vi "combinate.vi"(8 "error in (no error)":errorcluster caption="错误输入（无错误）", 11 "HJ212 输入":refnum<class "HJ212.lvclass">) -> (0 "error out":errorcluster caption="错误输出", 3 "HJ212 输出":refnum<class "HJ212.lvclass">)   [LabVIEW 2016, in "中水三立SQL数据传输.lvlib" / "HJ212.lvclass"]
uses:
  HJ212.lvclass
  data_combination/data_combination.lvclass/data_combination.ctl
  data_combination/data_combination.lvclass
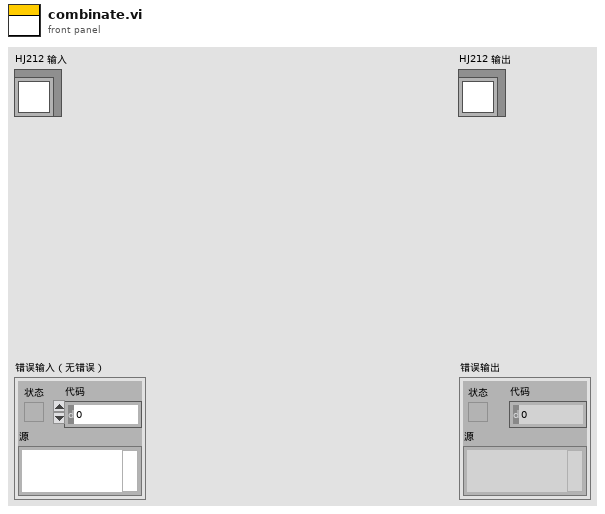
[diagram p1: front panel]
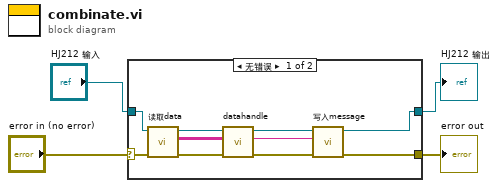
[diagram p0: block diagram]
diagram:
  n1 = case shown="无错误" "error in (no error)" {
    selector: "error in (no error)" -> [w12 w16]
    tunnel: "HJ212 输入" -> [w14 w15]
    tunnel: [w11 w16] -> w2
    tunnel: [w13 w15] -> w1
    frame No Error {
      n2 = call "读取data.vi"("error in (no error)"=w12, "data_combination输入"=w14) -> ("error out"=w6:errorcluster, "data"=w10:string[][], "data_combination输出"=w9:refnum<class "HJ212.lvclass">)  [unwired: 7 in]
      n3 = call-dynamic "datahandle.vi"("error in (no error)"=w6, "data"=w10, "HJ212 输入"=w9) -> ("error out"=w5:errorcluster, "message"=w7:string, "HJ212 输出"=w8:refnum<class "HJ212.lvclass">)  [unwired: 6 in]
      n4 = call "写入message.vi"("error in (no error)"=w5, "message"=w7, "data_combination输入"=w8) -> ("error out"=w11:errorcluster, "data_combination输出"=w13:refnum<class "HJ212.lvclass">)  [unwired: 7 in]
    }
    frame Error {
    }
  }
  "error out" <- w2
  "HJ212 输出" <- w1
